vi "ElevatorPresets.vi"(10 "Preset positions":T1, 11 "All Arduino Buttons":bool[](array[boolean])) -> ()   [LabVIEW 2014]
uses:
  PresetValues.ctl
  <vilib>/Rock Robotics/Network Tables/SD Write Number.vi
  <vilib>/Rock Robotics/Network Tables/SD Write Boolean.vi
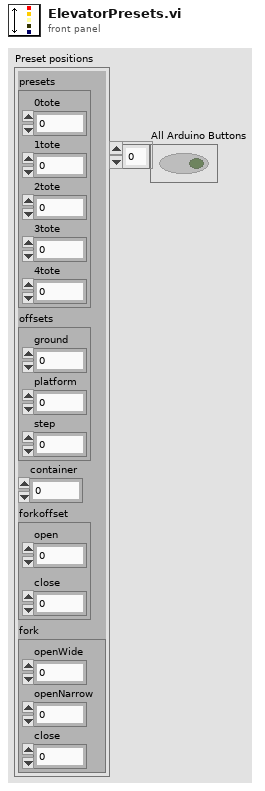
[diagram p1: front panel]
types:
  T1 = typedef "PresetValues.ctl" = cluster{"presets":cluster{"0tote":dbl, "1tote":dbl, "2tote":dbl, "3tote":dbl, "4tote":dbl}, "offsets":cluster{"ground":dbl, "platform":dbl, "step":dbl}, "container":dbl, "forkoffset":cluster{"open":dbl, "close":dbl}, "fork":cluster{"openWide":dbl, "openNarrow":dbl, "close":dbl}}
  T2 = cluster{"0tote":dbl, "1tote":dbl, "2tote":dbl, "3tote":dbl, "4tote":dbl}
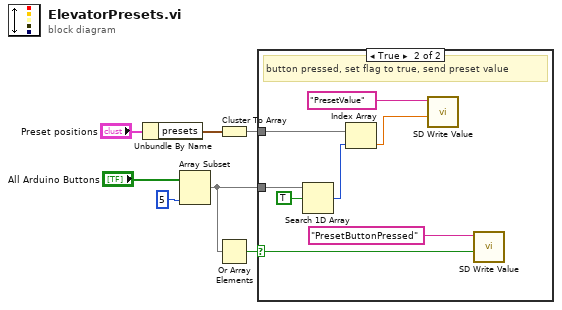
[diagram p0: block diagram]
diagram:
  n1 = Unbundle By Name("Preset positions") -> ("presets"=w1:T2)
  n2 = Array Subset(array="All Arduino Buttons", length=5) -> (w5:bool[])  [unwired: 1 in]
  n3 = Cluster To Array(cluster=w1) -> (array=w7:dbl[])
  n4 = Or Array Elements(Boolean array=w5) -> (logical OR=w4:bool)
  n5 = case shown="True" w4 {
    selector: w4 -> [_ w9]
    tunnel: w5 -> [_ w14]
    tunnel: w7 -> [_ w8]
    frame False {
      # "no button pressed, do nothing"
    }
    frame True {
      # "button pressed, set flag to true, send preset value"
      n6 = Search 1D Array(1D array=w14, element=TRUE) -> (index of element=w12:i32)  [unwired: 1 in]
      n7 = Index Array(array=w8, index=w12) -> (element=w11:dbl)
      n8 = call-poly <vilib>:"SD Write Value.vi"("Numeric"=w11, "Name"="PresetValue") -> ()  [unwired: 8 in, 2 out]
      n9 = call-poly <vilib>:"SD Write Value.vi"("Boolean"=w9, "Name"="PresetButtonPressed") -> ()  [unwired: 8 in, 2 out]
    }
  }
